vi "rsidr_core_global.vi"() -> ()   [LabVIEW 2020, in "Rohde&Schwarz RTx Oscilloscopes.lvlib"] (continued)
 "Access"=0, "Range Table"="", "Read Callback"="", "Write Callback"="", "Supported Models"="", "Instrument Options"="", "Flags"=0, "Help"="Return the time of the first sample of the indicated waveform.\n\nAvailable Repeated Capabilities:\nChannel: CH0, CH1, CH2, CH3, CH4, CHExt\r\n\nRemote-control command(s):\nCHANnel<m>:DATA:ENVelope:XORigin?"}, {"Level"=3, "Class Only"=FALSE, "Identifier"="RSRTX_ATTR_ENVELOPE_WAVEFORM_CONVERSION_X_INCREMENT", "Descriptive Name"="Envelope Waveform Conversion X Increment", "Data Type"=1, "Command"="CHAN{Channel}:DATA:ENV:XINC?", "Access"=0, "Range Table"="", "Read Callback"="", "Write Callback"="", "Supported Models"="", "Instrument Options"="", "Flags"=0, "Help"="Return the time difference between two adjacent samples of the indicated waveform.\n\nAvailable Repeated Capabilities:\nChannel: CH0, CH1, CH2, CH3, CH4, CHExt\r\n\nRemote-control command(s):\nCHANnel<m>:DATA:ENVelope:XINCrement?"}, {"Level"=3, "Class Only"=FALSE, "Identifier"="RSRTX_ATTR_ENVELOPE_WAVEFORM_CONVERSION_Y_START", "Descriptive Name"="Envelope Waveform Conversion Y Start", "Data Type"=1, "Command"="CHAN{Channel}:DATA:ENV:YOR?", "Access"=0, "Range Table"="", "Read Callback"="", "Write Callback"="", "Supported Models"="", "Instrument Options"="", "Flags"=0, "Help"="Return the voltage value for binary value 0 of the indicated waveform.\n\nAvailable Repeated Capabilities:\nChannel: CH0, CH1, CH2, CH3, CH4, CHExt\r\n\nRemote-control command(s):\nCHANnel<m>:DATA:ENVelope:YORigin?"}, {"Level"=3, "Class Only"=FALSE, "Identifier"="RSRTX_ATTR_ENVELOPE_WAVEFORM_CONVERSION_Y_INCREMENT", "Descriptive Name"="Envelope Waveform Conversion Y Increment", "Data Type"=1, "Command"="CHAN{Channel}:DATA:ENV:YINC?", "Access"=0, "Range Table"="", "Read Callback"="", "Write Callback"="", "Supported Models"="", "Instrument Options"="", "Flags"=0, "Help"="Return the voltage value per bit of the indicated waveform.\n\nAvailable Repeated Capabilities:\nChannel: CH0, CH1, CH2, CH3, CH4, CHExt\r\n\nRemote-control command(s):\nCHANnel<m>:DATA:ENVelope:YINCrement?"}, {"Level"=3, "Class Only"=FALSE, "Identifier"="RSRTX_ATTR_ENVELOPE_WAVEFORM_CONVERSION_Y_RESOLUTION", "Descriptive Name"="Envelope Waveform Conversion Y Resolution", "Data Type"=0, "Command"="CHAN{Channel}:DATA:ENV:YRES?", "Access"=0, "Range Table"="", "Read Callback"="", "Write Callback"="", "Supported Models"="", "Instrument Options"="", "Flags"=0, "Help"="Return the vertical bit resolution of the indicated waveform.\n\nAvailable Repeated Capabilities:\nChannel: CH0, CH1, CH2, CH3, CH4, CHExt\r\n\nRemote-control command(s):\nCHANnel<m>:DATA:ENVelope:YRESolution?"}, {"Level"=2, "Class Only"=TRUE, "Identifier"="", "Descriptive Name"="Math Waveform", "Data Type"=0, "Command"="", "Access"=0, "Range Table"="", "Read Callback"="", "Write Callback"="", "Supported Models"="", "Instrument Options"="", "Flags"=0, "Help"="Acquires waveform data."}, {"Level"=2, "Class Only"=TRUE, "Identifier"="", "Descriptive Name"="Math Waveform Conversion", "Data Type"=0, "Command"="", "Access"=0, "Range Table"="", "Read Callback"="", "Write Callback"="", "Supported Models"="", "Instrument Options"="", "Flags"=0, "Help"="Attributes for conversion of math waveform data."}, {"Level"=3, "Class Only"=FALSE, "Identifier"="RSRTX_ATTR_MATH_WAVEFORM_CONVERSION_X_START", "Descriptive Name"="Math Waveform Conversion X Start", "Data Type"=1, "Command"="CALC:MATH{Math}:DATA:XOR?", "Access"=0, "Range Table"="", "Read Callback"="", "Write Callback"="", "Supported Models"="RTM|RTA", "Instrument Options"="", "Flags"=0, "Help"="Return the time of the first sample of the indicated waveform.\n\nAvailable Repeated Capabilities:\nMath: MA1, MA2, MA3, MA4, MA5\r\n\nRemote-control command(s):\nCALCulate:MATH<m>:DATA:XORigin?"}, {"Level"=3, "Class Only"=FALSE, "Identifier"="RSRTX_ATTR_MATH_WAVEFORM_CONVERSION_X_INCREMENT", "Descriptive Name"="Math Waveform Conversion X Increment", "Data Type"=1, "Command"="CALC:MATH{Math}:DATA:XINC?", "Access"=0, "Range Table"="", "Read Callback"="", "Write Callback"="", "Supported Models"="RTM|RTA", "Instrument Options"="", "Flags"=0, "Help"="Return the time difference between two adjacent samples of the indicated waveform.\n\nAvailable Repeated Capabilities:\nMath: MA1, MA2, MA3, MA4, MA5\r\n\nRemote-control command(s):\nCALCulate:MATH<m>:DATA:XINCrement?"}, {"Level"=3, "Class Only"=FALSE, "Identifier"="RSRTX_ATTR_MATH_WAVEFORM_CONVERSION_Y_START", "Descriptive Name"="Math Waveform Conversion Y Start", "Data Type"=1, "Command"="CALC:MATH{Math}:DATA:YOR?", "Access"=0, "Range Table"="", "Read Callback"="", "Write Callback"="", "Supported Models"="RTM|RTA", "Instrument Options"="", "Flags"=0, "Help"="Return the voltage value for binary value 0 of the indicated waveform.\n\nAvailable Repeated Capabilities:\nMath: MA1, MA2, MA3, MA4, MA5\r\n\nRemote-control command(s):\nCALCulate:MATH<m>:DATA:YORigin?"}, {"Level"=3, "Class Only"=FALSE, "Identifier"="RSRTX_ATTR_MATH_WAVEFORM_CONVERSION_Y_INCREMENT", "Descriptive Name"="Math Waveform Conversion Y Increment", "Data Type"=1, "Command"="CALC:MATH{Math}:DATA:YINC?", "Access"=0, "Range Table"="", "Read Callback"="", "Write Callback"="", "Supported Models"="RTM|RTA", "Instrument Options"="", "Flags"=0, "Help"="Return the voltage value per bit of the indicated waveform.\n\nAvailable Repeated Capabilities:\nMath: MA1, MA2, MA3, MA4, MA5\r\n\nRemote-control command(s):\nCALCulate:MATH<m>:DATA:YINCrement?"}, {"Level"=3, "Class Only"=FALSE, "Identifier"="RSRTX_ATTR_MATH_WAVEFORM_CONVERSION_Y_RESOLUTION", "Descriptive Name"="Math Waveform Conversion Y Resolution", "Data Type"=0, "Command"="CALC:MATH{Math}:DATA:YRES?", "Access"=0, "Range Table"="", "Read Callback"="", "Write Callback"="", "Supported Models"="RTM|RTA", "Instrument Options"="", "Flags"=0, "Help"="Return the vertical bit resolution of the indicated waveform.\n\nAvailable Repeated Capabilities:\nMath: MA1, MA2, MA3, MA4, MA5\r\n\nRemote-control command(s):\nCALCulate:MATH<m>:DATA:YRESolution?"}, {"Level"=2, "Class Only"=TRUE, "Identifier"="", "Descriptive Name"="Simple Math Waveform (RTB)", "Data Type"=0, "Command"="", "Access"=0, "Range Table"="", "Read Callback"="", "Write Callback"="", "Supported Models"="", "Instrument Options"="", "Flags"=0, "Help"="Acquires waveform data."}, {"Level"=2, "Class Only"=TRUE, "Identifier"="", "Descriptive Name"="Simple Math Waveform Conversion (RTB)", "Data Type"=0, "Command"="", "Access"=0, "Range Table"="", "Read Callback"="", "Write Callback"="", "Supported Models"="", "Instrument Options"="", "Flags"=0, "Help"="Attributes for conversion of math waveform data."}, {"Level"=3, "Class Only"=FALSE, "Identifier"="RSRTX_ATTR_SIMPLE_MATH_WAVEFORM_CONVERSION_X_START", "Descriptive Name"="Simple Math Waveform Conversion X Start", "Data Type"=1, "Command"="CALC:QMAT:DATA:XOR?", "Access"=0, "Range Table"="", "Read Callback"="", "Write Callback"="", "Supported Models"="RTB", "Instrument Options"="", "Flags"=0, "Help"="Return the time of the first sample of the indicated waveform.\n\nAvailable Repeated Capabilities:\nNone\n\nRemote-control command(s):\nCALCulate:QMATh:DATA:XORigin?"}, {"Level"=3, "Class Only"=FALSE, "Identifier"="RSRTX_ATTR_SIMPLE_MATH_WAVEFORM_CONVERSION_X_INCREMENT", "Descriptive Name"="Simple Math Waveform Conversion X Increment", "Data Type"=1, "Command"="CALC:QMAT:DATA:XINC?", "Access"=0, "Range Table"="", "Read Callback"="", "Write Callback"="", "Supported Models"="RTB", "Instrument Options"="", "Flags"=0, "Help"="Return the time difference between two adjacent samples of the indicated waveform.\n\nAvailable Repeated Capabilities:\nNone\n\nRemote-control command(s):\nCALCulate:QMATh:DATA:XINCrement?"}, {"Level"=3, "Class Only"=FALSE, "Identifier"="RSRTX_ATTR_SIMPLE_MATH_WAVEFORM_CONVERSION_Y_START", "Descriptive Name"="Simple Math Waveform Conversion Y Start", "Data Type"=1, "Command"="CALC:QMAT:DATA:YOR?", "Access"=0, "Range Table"="", "Read Callback"="", "Write Callback"="", "Supported Models"="RTB", "Instrument Options"="", "Flags"=0, "Help"="Return the voltage value for binary value 0 of the indicated waveform.\n\nAvailable Repeated Capabilities:\nNone\n\nRemote-control command(s):\nCALCulate:QMATh:DATA:YORigin?"}, {"Level"=3, "Class Only"=FALSE, "Identifier"="RSRTX_ATTR_SIMPLE_MATH_WAVEFORM_CONVERSION_Y_INCREMENT", "Descriptive Name"="Simple Math Waveform Conversion Y Increment", "Data Type"=1, "Command"="CALC:QMAT:DATA:YINC?", "Access"=0, "Range Table"="", "Read Callback"="", "Write Callback"="", "Supported Models"="RTB", "Instrument Options"="", "Flags"=0, "Help"="Return the voltage value per bit of the indicated waveform.\n\nAvailable Repeated Capabilities:\nNone\n\nRemote-control command(s):\nCALCulate:QMATh:DATA:YINCrement?"}, {"Level"=3, "Class Only"=FALSE, "Identifier"="RSRTX_ATTR_SIMPLE_MATH_WAVEFORM_CONVERSION_Y_RESOLUTION", "Descriptive Name"="Simple Math Waveform Conversion Y Resolution", "Data Type"=0, "Command"="CALC:QMAT:DATA:YRES?", "Access"=0, "Range Table"="", "Read Callback"="", "Write Callback"="", "Supported Models"="RTB", "Instrument Options"="", "Flags"=0, "Help"="Return the vertical bit resolution of the indicated waveform.\n\nAvailable Repeated Capabilities:\nNone\n\nRemote-control command(s):\nCALCulate:QMATh:DATA:YRESolution?"}, {"Level"=2, "Class Only"=TRUE, "Identifier"="", "Descriptive Name"="Reference Waveform", "Data Type"=0, "Command"="", "Access"=0, "Range Table"="", "Read Callback"="", "Write Callback"="", "Supported Models"="", "Instrument Options"="", "Flags"=0, "Help"="Acquires waveform data."}, {"Level"=2, "Class Only"=TRUE, "Identifier"="", "Descriptive Name"="Reference Waveform Conversion", "Data Type"=0, "Command"="", "Access"=0, "Range Table"="", "Read Callback"="", "Write Callback"="", "Supported Models"="", "Instrument Options"="", "Flags"=0, "Help"="Attributes for conversion of reference waveform data."}, {"Level"=3, "Class Only"=FALSE, "Identifier"="RSRTX_ATTR_REFERENCE_WAVEFORM_CONVERSION_X_START", "Descriptive Name"="Reference Waveform Conversion X Start", "Data Type"=1, "Command"="REFC{ReferenceWfm}:DATA:XOR?", "Access"=0, "Range Table"="", "Read Callback"="", "Write Callback"="", "Supported Models"="", "Instrument Options"="", "Flags"=0, "Help"="Return the time of the first sample of the indicated waveform.\n\nAvailable Repeated Capabilities:\nReferenceWfm: RW1, RW2, RW3, RW4\r\n\nRemote-control command(s):\nREFCurvel<m>:DATA:XORigin?"}, {"Level"=3, "Class Only"=FALSE, "Identifier"="RSRTX_ATTR_REFERENCE_WAVEFORM_CONVERSION_X_INCREMENT", "Descriptive Name"="Reference Waveform Conversion X Increment", "Data Type"=1, "Command"="REFC{ReferenceWfm}:DATA:XINC?", "Access"=0, "Range Table"="", "Read Callback"="", "Write Callback"="", "Supported Models"="", "Instrument Options"="", "Flags"=0, "Help"="Return the time difference between two adjacent samples of the indicated waveform.\n\nAvailable Repeated Capabilities:\nReferenceWfm: RW1, RW2, RW3, RW4\r\n\nRemote-control command(s):\nREFCurve<m>:DATA:XINCrement?"}, {"Level"=3, "Class Only"=FALSE, "Identifier"="RSRTX_ATTR_REFERENCE_WAVEFORM_CONVERSION_Y_START", "Descriptive Name"="Reference Waveform Conversion Y Start", "Data Type"=1, "Command"="REFC{ReferenceWfm}:DATA:YOR?", "Access"=0, "Range Table"="", "Read Callback"="", "Write Callback"="", "Supported Models"="", "Instrument Options"="", "Flags"=0, "Help"="Return the voltage value for binary value 0 of the indicated waveform.\n\nAvailable Repeated Capabilities:\nReferenceWfm: RW1, RW2, RW3, RW4\r\n\nRemote-control command(s):\nREFCurve<m>:DATA:YORigin?"}, {"Level"=3, "Class Only"=FALSE, "Identifier"="RSRTX_ATTR_REFERENCE_WAVEFORM_CONVERSION_Y_INCREMENT", "Descriptive Name"="Reference Waveform Conversion Y Increment", "Data Type"=1, "Command"="REFC{ReferenceWfm}:DATA:YINC?", "Access"=0, "Range Table"="", "Read Callback"="", "Write Callback"="", "Supported Models"="", "Instrument Options"="", "Flags"=0, "Help"="Return the voltage value per bit of the indicated waveform.\n\nAvailable Repeated Capabilities:\nReferenceWfm: RW1, RW2, RW3, RW4\r\n\nRemote-control command(s):\nREFCurve<m>:DATA:YINCrement?"}, {"Level"=3, "Class Only"=FALSE, "Identifier"="RSRTX_ATTR_REFERENCE_WAVEFORM_CONVERSION_Y_RESOLUTION", "Descriptive Name"="Reference Waveform Conversion Y Resolution", "Data Type"=0, "Command"="REFC{ReferenceWfm}:DATA:YRES?", "Access"=0, "Range Table"="", "Read Callback"="", "Write Callback"="", "Supported Models"="", "Instrument Options"="", "Flags"=0, "Help"="Return the vertical bit resolution of the indicated waveform.\n\nAvailable Repeated Capabilities:\nReferenceWfm: RW1, RW2, RW3, RW4\r\n\nRemote-control command(s):\nREFCurve<m>:DATA:YRESolution?"}, {"Level"=2, "Class Only"=TRUE, "Identifier"="", "Descriptive Name"="Mask Data", "Data Type"=0, "Command"="", "Access"=0, "Range Table"="", "Read Callback"="", "Write Callback"="", "Supported Models"="", "Instrument Options"="", "Flags"=0, "Help"="Acquires mask data."}, {"Level"=2, "Class Only"=TRUE, "Identifier"="", "Descriptive Name"="Mask Data Conversion", "Data Type"=0, "Command"="", "Access"=0, "Range Table"="", "Read Callback"="", "Write Callback"="", "Supported Models"="", "Instrument Options"="", "Flags"=0, "Help"="Attributes for conversion of mask data."}, {"Level"=3, "Class Only"=FALSE, "Identifier"="RSRTX_ATTR_MASK_DATA_CONVERSION_X_START", "Descriptive Name"="Mask Data Conversion X Start", "Data Type"=1, "Command"="MASK:DATA:XOR?", "Access"=0, "Range Table"="", "Read Callback"="", "Write Callback"="", "Supported Models"="", "Instrument Options"="", "Flags"=0, "Help"="Return the time of the first sample of the indicated waveform.\n\nAvailable Repeated Capabilities:\nNone\n\nRemote-control command(s):\nMASK:DATA:XORigin?"}, {"Level"=3, "Class Only"=FALSE, "Identifier"="RSRTX_ATTR_MASK_DATA_CONVERSION_X_INCREMENT", "Descriptive Name"="Mask Data Conversion X Increment", "Data Type"=1, "Command"="MASK:DATA:XINC?", "Access"=0, "Range Table"="", "Read Callback"="", "Write Callback"="", "Supported Models"="", "Instrument Options"="", "Flags"=0, "Help"="Return the time difference between two adjacent samples of the indicated waveform.\n\nAvailable Repeated Capabilities:\nNone\n\nRemote-control command(s):\nMASK:DATA:XINCrement?"}, {"Level"=3, "Class Only"=FALSE, "Identifier"="RSRTX_ATTR_MASK_DATA_CONVERSION_Y_START", "Descriptive Name"="Mask Data Conversion Y Start", "Data Type"=1, "Command"="MASK:DATA:YOR?", "Access"=0, "Range Table"="", "Read Callback"="", "Write Callback"="", "Supported Models"="", "Instrument Options"="", "Flags"=0, "Help"="Return the voltage value for binary value 0 of the indicated waveform.\n\nAvailable Repeated Capabilities:\nNone\n\nRemote-control command(s):\nMASK:DATA:YORigin?"}, {"Level"=3, "Class Only"=FALSE, "Identifier"="RSRTX_ATTR_MASK_DATA_CONVERSION_Y_INCREMENT", "Descriptive Name"="Mask Data Conversion Y Increment", "Data Type"=1, "Command"="MASK:DATA:YINC?", "Access"=0, "Range Table"="", "Read Callback"="", "Write Callback"="", "Supported Models"="", "Instrument Options"="", "Flags"=0, "Help"="Return the voltage value per bit of the indicated waveform.\n\nAvailable Repeated Capabilities:\nNone\n\nRemote-control command(s):\nMASK:DATA:YINCrement?"}, {"Level"=3, "Class Only"=FALSE, "Identifier"="RSRTX_ATTR_MASK_DATA_CONVERSION_Y_RESOLUTION", "Descriptive Name"="Mask Data Conversion Y Resolution", "Data Type"=0, "Command"="MASK:DATA:YRES?", "Access"=0, "Range Table"="", "Read Callback"="", "Write Callback"="", "Supported Models"="", "Instrument Options"="", "Flags"=0, "Help"="Return the vertical bit resolution of the indicated waveform.\n\nAvailable Repeated Capabilities:\nNone\n\nRemote-control command(s):\nMASK:DATA:YRESolution?"}, {"Level"=2, "Class Only"=TRUE, "Identifier"="", "Descriptive Name"="Logic Data", "Data Type"=0, "Command"="", "Access"=0, "Range Table"="", "Read Callback"="", "Write Callback"="", "Supported Models"="", "Instrument Options"="", "Flags"=0, "Help"="Acquires logic data."}, {"Level"=2, "Class Only"=TRUE, "Identifier"="", "Descriptive Name"="Logic Data Conversion", "Data Type"=0, "Command"="", "Access"=0, "Range Table"="", "Read Callback"="", "Write Callback"="", "Supported Models"="", "Instrument Options"="", "Flags"=0, "Help"="Attributes for conversion of logic data."}, {"Level"=3, "Class Only"=FALSE, "Identifier"="RSRTX_ATTR_LOGIC_DATA_CONVERSION_X_START", "Descriptive Name"="Logic Data Conversion X Start", "Data Type"=1, "Command"="LOG{Logic}:DATA:XOR?", "Access"=0, "Range Table"="", "Read Callback"="", "Write Callback"="", "Supported Models"="", "Instrument Options"="", "Flags"=0, "Help"="Return the time of the first sample of the indicated waveform.\n\nAvailable Repeated Capabilities:\nLogic: Logic1, Logic2\r\n\nRemote-control command(s):\nLOGic<p>:DATA:XORigin?"}, {"Level"=3, "Class Only"=FALSE, "Identifier"="RSRTX_ATTR_LOGIC_DATA_CONVERSION_X_INCREMENT", "Descriptive Name"="Logic Data Conversion X Increment", "Data Type"=1, "Command"="LOG{Logic}:DATA:XINC?", "Access"=0, "Range Table"="", "Read Callback"="", "Write Callback"="", "Supported Models"="", "Instrument Options"="", "Flags"=0, "Help"="Return the time difference between two adjacent samples of the indicated waveform.\n\nAvailable Repeated Capabilities:\nLogic: Logic1, Logic2\r\n\nRemote-control command(s):\nLOGic<p>:DATA:XINCrement?"}, {"Level"=3, "Class Only"=FALSE, "Identifier"="RSRTX_ATTR_LOGIC_DATA_CONVERSION_Y_START", "Descriptive Name"="Logic Data Conversion Y Start", "Data Type"=1, "Command"="LOG{Logic}:DATA:YOR?", "Access"=0, "Range Table"="", "Read Callback"="", "Write Callback"="", "Supported Models"="", "Instrument Options"="", "Flags"=0, "Help"="Return the voltage value for binary value 0 of the indicated waveform.\n\nAvailable Repeated Capabilities:\nLogic: Logic1, Logic2\r\n\nRemote-control command(s):\nLOGic<p>:DATA:YORigin?"}, {"Level"=3, "Class Only"=FALSE, "Identifier"="RSRTX_ATTR_LOGIC_DATA_CONVERSION_Y_INCREMENT", "Descriptive Name"="Logic Data Conversion Y Increment", "Data Type"=1, "Command"="LOG{Logic}:DATA:YINC?", "Access"=0, "Range Table"="", "Read Callback"="", "Write Callback"="", "Supported Models"="", "Instrument Options"="", "Flags"=0, "Help"="Return the voltage value per bit of the indicated waveform.\n\nAvailable Repeated Capabilities:\nLogic: Logic1, Logic2\r\n\nRemote-control command(s):\nLOGic<p>:DATA:YINCrement?"}, {"Level"=3, "Class Only"=FALSE, "Identifier"="RSRTX_ATTR_LOGIC_DATA_CONVERSION_Y_RESOLUTION", "Descriptive Name"="Logic Data Conversion Y Resolution", "Data Type"=0, "Command"="LOG{Logic}:DATA:YRES?", "Access"=0, "Range Table"="", "Read Callback"="", "Write Callback"="", "Supported Models"="", "Instrument Options"="", "Flags"=0, "Help"="Return the vertical bit resolution of the indicated waveform.\n\nAvailable Repeated Capabilities:\nLogic: Logic1, Logic2\r\n\nRemote-control command(s):\nLOGic<p>:DATA:YRESolution?"}, {"Level"=2, "Class Only"=TRUE, "Identifier"="", "Descriptive Name"="Digital Data", "Data Type"=0, "Command"="", "Access"=0, "Range Table"="", "Read Callback"="", "Write Callback"="", "Supported Models"="", "Instrument Options"="", "Flags"=0, "Help"="Acquires digital data."}, {"Level"=3, "Class Only"=FALSE, "Identifier"="RSRTX_ATTR_DIGITAL_WAVEFORM_SAMPLES", "Descriptive Name"="Digital Waveform Samples", "Data Type"=0, "Command"="DIG{Digital}:DATA:POIN?", "Access"=0, "Range Table"="", "Read Callback"="", "Write Callback"="", "Supported Models"="", "Instrument Options"="", "Flags"=0, "Help"="Returns the number of returned samples for the selected range.\n\nAvailable Repeated Capabilities:\nDigital: D0, D1, D2, D3, D4, D5, D6, D7, D8, D9, D10, D11, D12, D13, D14, D15\r\n\nRemote-control command(s):\nDIGital<m>:DATA:POINts?"}, {"Level"=2, "Class Only"=TRUE, "Identifier"="", "Descriptive Name"="Digital Data Conversion", "Data Type"=0, "Command"="", "Access"=0, "Range Table"="", "Read Callback"="", "Write Callback"="", "Supported Models"="", "Instrument Options"="", "Flags"=0, "Help"="Attributes for conversion of digital data."}, {"Level"=3, "Class Only"=FALSE, "Identifier"="RSRTX_ATTR_DIGITAL_DATA_CONVERSION_X_START", "Descriptive Name"="Digital Data Conversion X Start", "Data Type"=1, "Command"="DIG{Digital}:DATA:XOR?", "Access"=0, "Range Table"="", "Read Callback"="", "Write Callback"="", "Supported Models"="", "Instrument Options"="", "Flags"=0, "Help"="Return the time of the first sample of the indicated waveform.\n\nAvailable Repeated Capabilities:\nDigital: D0, D1, D2, D3, D4, D5, D6, D7, D8, D9, D10, D11, D12, D13, D14, D15\r\n\nRemote-control command(s):\nDIGital<m>:DATA:XORigin?"}, {"Level"=3, "Class Only"=FALSE, "Identifier"="RSRTX_ATTR_DIGITAL_DATA_CONVERSION_X_INCREMENT", "Descriptive Name"="Digital Data Conversion X Increment", "Data Type"=1, "Command"="DIG{Digital}:DATA:XINC?", "Access"=0, "Range Table"="", "Read Callback"="", "Write Callback"="", "Supported Models"="", "Instrument Options"="", "Flags"=0, "Help"="Return the time difference between two adjacent samples of the indicated waveform.\n\nAvailable Repeated Capabilities:\nDigital: D0, D1, D2, D3, D4, D5, D6, D7, D8, D9, D10, D11, D12, D13, D14, D15\r\n\nRemote-control command(s):\nDIGital<m>:DATA:XINCrement?"}, {"Level"=3, "Class Only"=FALSE, "Identifier"="RSRTX_ATTR_DIGITAL_DATA_CONVERSION_Y_START", "Descriptive Name"="Digital Data Conversion Y Start", "Data Type"=1, "Command"="DIG{Digital}:DATA:YOR?", "Access"=0, "Range Table"="", "Read Callback"="", "Write Callback"="", "Supported Models"="", "Instrument Options"="", "Flags"=0, "Help"="Return the voltage value for binary value 0 of the indicated waveform.\n\nAvailable Repeated Capabilities:\nDigital: D0, D1, D2, D3, D4, D5, D6, D7, D8, D9, D10, D11, D12, D13, D14, D15\r\n\nRemote-control command(s):\nDIGital<m>:DATA:YORigin?"}, {"Level"=3, "Class Only"=FALSE, "Identifier"="RSRTX_ATTR_DIGITAL_DATA_CONVERSION_Y_INCREMENT", "Descriptive Name"="Digital Data Conversion Y Increment", "Data Type"=1, "Command"="DIG{Digital}:DATA:YINC?", "Access"=0, "Range Table"="", "Read Callback"="", "Write Callback"="", "Supported Models"="", "Instrument Options"="", "Flags"=0, "Help"="Return the voltage value per bit of the indicated waveform.\n\nAvailable Repeated Capabilities:\nDigital: D0, D1, D2, D3, D4, D5, D6, D7, D8, D9, D10, D11, D12, D13, D14, D15\r\n\nRemote-control command(s):\nDIGital<m>:DATA:YINCrement?"}, {"Level"=3, "Class Only"=FALSE, "Identifier"="RSRTX_ATTR_DIGITAL_DATA_CONVERSION_Y_RESOLUTION", "Descriptive Name"="Digital Data Conversion Y Resolution", "Data Type"=0, "Command"="DIG{Digital}:DATA:YRES?", "Access"=0, "Range Table"="", "Read Callback"="", "Write Callback"="", "Supported Models"="", "Instrument Options"="", "Flags"=0, "Help"="Return the vertical bit resolution of the indicated waveform.\n\nAvailable Repeated Capabilities:\nDigital: D0, D1, D2, D3, D4, D5, D6, D7, D8, D9, D10, D11, D12, D13, D14, D15\r\n\nRemote-control command(s):\nDIGital<m>:DATA:YRESolution?"}, {"Level"=2, "Class Only"=TRUE, "Identifier"="", "Descriptive Name"="Spectrum Data", "Data Type"=0, "Command"="", "Access"=0, "Range Table"="", "Read Callback"="", "Write Callback"="", "Supported Models"="", "Instrument Options"="", "Flags"=0, "Help"="Acquires spectrum data."}, {"Level"=3, "Class Only"=FALSE, "Identifier"="RSRTX_ATTR_SPECTRUM_WAVEFORM_SAMPLES", "Descriptive Name"="Spectrum Waveform Samples", "Data Type"=0, "Command"="SPEC:WAV:SPEC:DATA:POIN?", "Access"=0, "Range Table"="", "Read Callback"="", "Write Callback"="", "Supported Models"="", "Instrument Options"="", "Flags"=0, "Help"="Returns the number of data samples that are returned with SPECtrum:WAVeform:SPECtrum:DATA.\n\nAvailable Repeated Capabilities:\nNone\n\nRemote-control command(s):\nSPECtrum:WAVeform:SPECtrum:DATA:POINts?"}, {"Level"=3, "Class Only"=TRUE, "Identifier"="", "Descriptive Name"="Minimum", "Data Type"=0, "Command"="", "Access"=0, "Range Table"="", "Read Callback"="", "Write Callback"="", "Supported Models"="", "Instrument Options"="", "Flags"=0, "Help"="Acquires spectrum minimum data."}, {"Level"=4, "Class Only"=FALSE, "Identifier"="RSRTX_ATTR_SPECTRUM_MINIMUM_WAVEFORM_SAMPLES", "Descriptive Name"="Spectrum Minimum Waveform Samples", "Data Type"=0, "Command"="SPEC:WAV:MIN:DATA:POIN?", "Access"=0, "Range Table"="", "Read Callback"="", "Write Callback"="", "Supported Models"="", "Instrument Options"="", "Flags"=0, "Help"="Returns the number of data samples that are returned with SPECtrum:WAVeform:MINimum:DATA.\n\nAvailable Repeated Capabilities:\nNone\n\nRemote-control command(s):\nSPECtrum:WAVeform:MINimum:DATA:POINts?"}, {"Level"=3, "Class Only"=TRUE, "Identifier"="", "Descriptive Name"="Maximum", "Data Type"=0, "Command"="", "Access"=0, "Range Table"="", "Read Callback"="", "Write Callback"="", "Supported Models"="", "Instrument Options"="", "Flags"=0, "Help"="Acquires spectrum maximum data."}, {"Level"=4, "Class Only"=FALSE, "Identifier"="RSRTX_ATTR_SPECTRUM_MAXIMUM_WAVEFORM_SAMPLES", "Descriptive Name"="Spectrum Maximum Waveform Samples", "Data Type"=0, "Command"="SPEC:WAV:MAX:DATA:POIN?", "Access"=0, "Range Table"="", "Read Callback"="", "Write Callback"="", "Supported Models"="", "Instrument Options"="", "Flags"=0, "Help"="Returns the number of data samples that are returned with SPECtrum:WAVeform:xxx:DATA for the indicated waveform.\n\nAvailable Repeated Capabilities:\nNone\n\nRemote-control command(s):\nSPECtrum:WAVeform:MAXimum:DATA:POINts?"}, {"Level"=3, "Class Only"=TRUE, "Identifier"="", "Descriptive Name"="Average", "Data Type"=0, "Command"="", "Access"=0, "Range Table"="", "Read Callback"="", "Write Callback"="", "Supported Models"="", "Instrument Options"="", "Flags"=0, "Help"="Acquires spectrum average data."}, {"Level"=4, "Class Only"=FALSE, "Identifier"="RSRTX_ATTR_SPECTRUM_AVERAGE_WAVEFORM_SAMPLES", "Descriptive Name"="Spectrum Average Waveform Samples", "Data Type"=0, "Command"="SPEC:WAV:AVER:DATA:POIN?", "Access"=0, "Range Table"="", "Read Callback"="", "Write Callback"="", "Supported Models"="", "Instrument Options"="", "Flags"=0, "Help"="Returns the number of data samples that are returned with SPECtrum:WAVeform:xxx:DATA for the indicated waveform.\n\nAvailable Repeated Capabilities:\nNone\n\nRemote-control command(s):\nSPECtrum:WAVeform:AVERage:DATA:POINts?"}, {"Level"=2, "Class Only"=TRUE, "Identifier"="", "Descriptive Name"="Spectrum Data Conversion", "Data Type"=0, "Command"="", "Access"=0, "Range Table"="", "Read Callback"="", "Write Callback"="", "Supported Models"="", "Instrument Options"="", "Flags"=0, "Help"="Attributes for conversion of spectrum data."}, {"Level"=3, "Class Only"=FALSE, "Identifier"="RSRTX_ATTR_SPECTRUM_DATA_CONVERSION_X_START", "Descriptive Name"="Spectrum Data Conversion X Start", "Data Type"=1, "Command"="SPEC:WAV:SPEC:DATA:XOR?", "Access"=0, "Range Table"="", "Read Callback"="", "Write Callback"="", "Supported Models"="", "Instrument Options"="", "Flags"=0, "Help"="Returns the frequency of the first sample of the indicated waveform.\n\nAvailable Repeated Capabilities:\nNone\n\nRemote-control command(s):\nSPECtrum:WAVeform:SPECtrum:DATA:XORigin?"}, {"Level"=3, "Class Only"=FALSE, "Identifier"="RSRTX_ATTR_SPECTRUM_DATA_CONVERSION_X_INCREMENT", "Descriptive Name"="Spectrum Data Conversion X Increment", "Data Type"=1, "Command"="SPEC:WAV:SPEC:DATA:XINC?", "Access"=0, "Range Table"="", "Read Callback"="", "Write Callback"="", "Supported Models"="", "Instrument Options"="", "Flags"=0, "Help"="Return the level difference between two adjacent samples of the indicated waveform.\n\nAvailable Repeated Capabilities:\nNone\n\nRemote-control command(s):\nSPECtrum:WAVeform:SPECtrum:DATA:XINCrement?"}, {"Level"=3, "Class Only"=FALSE, "Identifier"="RSRTX_ATTR_SPECTRUM_DATA_CONVERSION_Y_START", "Descriptive Name"="Spectrum Data Conversion Y Start", "Data Type"=1, "Command"="SPEC:WAV:SPEC:DATA:YOR?", "Access"=0, "Range Table"="", "Read Callback"="", "Write Callback"="", "Supported Models"="", "Instrument Options"="", "Flags"=0, "Help"="Returns the vertical bit resolution of the indicated waveform.\n\nAvailable Repeated Capabilities:\nNone\n\nRemote-control command(s):\nSPECtrum:WAVeform:SPECtrum:DATA:YORigin?"}, {"Level"=3, "Class Only"=FALSE, "Identifier"="RSRTX_ATTR_SPECTRUM_DATA_CONVERSION_Y_INCREMENT", "Descriptive Name"="Spectrum Data Conversion Y Increment", "Data Type"=1, "Command"="SPEC:WAV:SPEC:DATA:YINC?", "Access"=0, "Range Table"="", "Read Callback"="", "Write Callback"="", "Supported Models"="", "Instrument Options"="", "Flags"=0, "Help"="Returns the voltage value per bit of the indicated waveform.\n\nAvailable Repeated Capabilities:\nNone\n\nRemote-control command(s):\nSPECtrum:WAVeform:SPECtrum:DATA:YINCrement?"}, {"Level"=3, "Class Only"=FALSE, "Identifier"="RSRTX_ATTR_SPECTRUM_DATA_CONVERSION_Y_RESOLUTION", "Descriptive Name"="Spectrum Data Conversion Y Resolution", "Data Type"=0, "Command"="SPEC:WAV:SPEC:DATA:YRES?", "Access"=0, "Range Table"="", "Read Callback"="", "Write Callback"="", "Supported Models"="", "Instrument Options"="", "Flags"=0, "Help"="Returns the vertical bit resolution of the indicated waveform.\n\nAvailable Repeated Capabilities:\nNone\n\nRemote-control command(s):\nSPECtrum:WAVeform:SPECtrum:DATA:YRESolution?"}, {"Level"=3, "Class Only"=TRUE, "Identifier"="", "Descriptive Name"="Minimum", "Data Type"=0, "Command"="", "Access"=0, "Range Table"="", "Read Callback"="", "Write Callback"="", "Supported Models"="", "Instrument Options"="", "Flags"=0, "Help"="Attributes for conversion of spectrum minimum data."}, {"Level"=4, "Class Only"=FALSE, "Identifier"="RSRTX_ATTR_SPECTRUM_MINIMUM_DATA_CONVERSION_X_START", "Descriptive Name"="Spectrum Minimum Data Conversion X Start", "Data Type"=1, "Command"="SPEC:WAV:MIN:DATA:XOR?", "Access"=0, "Range Table"="", "Read Callback"="", "Write Callback"="", "Supported Models"="", "Instrument Options"="", "Flags"=0, "Help"="Returns the frequency of the first sample of the indicated waveform.\n\nAvailable Repeated Capabilities:\nNone\n\nRemote-control command(s):\nSPECtrum:WAVeform:MINimum:DATA:XORigin?"}, {"Level"=4, "Class Only"=FALSE, "Identifier"="RSRTX_ATTR_SPECTRUM_MINIMUM_DATA_CONVERSION_X_INCREMENT", "Descriptive Name"="Spectrum Minimum Data Conversion X Increment", "Data Type"=1, "Command"="SPEC:WAV:MIN:DATA:XINC?", "Access"=0, "Range Table"="", "Read Callback"="", "Write Callback"="", "Supported Models"="", "Instrument Options"="", "Flags"=0, "Help"="Return the level difference between two adjacent samples of the indicated waveform.\n\nAvailable Repeated Capabilities:\nNone\n\nRemote-control command(s):\nSPECtrum:WAVeform:MINimum:DATA:XINCrement?"}, {"Level"=4, "Class Only"=FALSE, "Identifier"="RSRTX_ATTR_SPECTRUM_MINIMUM_DATA_CONVERSION_Y_START", "Descriptive Name"="Spectrum Minimum Data Conversion Y Start", "Data Type"=1, "Command"="SPEC:WAV:MIN:DATA:YOR?", "Access"=0, "Range Table"="", "Read Callback"="", "Write Callback"="", "Supported Models"="", "Instrument Options"="", "Flags"=0, "Help"="Returns the vertical bit resolution of the indicated waveform.\n\nAvailable Repeated Capabilities:\nNone\n\nRemote-control command(s):\nSPECtrum:WAVeform:MINimum:DATA:YORigin?"}, {"Level"=4, "Class Only"=FALSE, "Identifier"="RSRTX_ATTR_SPECTRUM_MINIMUM_DATA_CONVERSION_Y_INCREMENT", "Descriptive Name"="Spectrum Minimum Data Conversion Y Increment", "Data Type"=1, "Command"="SPEC:WAV:MIN:DATA:YINC?", "Access"=0, "Range Table"="", "Read Callback"="", "Write Callback"="", "Supported Models"="", "Instrument Options"="", "Flags"=0, "Help"="Returns the voltage value per bit of the indicated waveform.\n\nAvailable Repeated Capabilities:\nNone\n\nRemote-control command(s):\nSPECtrum:WAVeform:MINimum:DATA:YINCrement?"}, {"Level"=4, "Class Only"=FALSE, "Identifier"="RSRTX_ATTR_SPECTRUM_MINIMUM_DATA_CONVERSION_Y_RESOLUTION", "Descriptive Name"="Spectrum Minimum Data Conversion Y Resolution", "Data Type"=0, "Command"="SPEC:WAV:MIN:DATA:YRES?", "Access"=0, "Range Table"="", "Read Callback"="", "Write Callback"="", "Supported Models"="", "Instrument Options"="", "Flags"=0, "Help"="Returns the vertical bit resolution of the indicated waveform.\n\nAvailable Repeated Capabilities:\nNone\n\nRemote-control command(s):\nSPECtrum:WAVeform:MINimum:DATA:YRESolution?"}, {"Level"=3, "Class Only"=TRUE, "Identifier"="", "Descriptive Name"="Maximum", "Data Type"=0, "Command"="", "Access"=0, "Range Table"="", "Read Callback"="", "Write Callback"="", "Supported Models"="", "Instrument Options"="", "Flags"=0, "Help"="Attributes for conversion of spectrum maximum data."}, {"Level"=4, "Class Only"=FALSE, "Identifier"="RSRTX_ATTR_SPECTRUM_MAXIMUM_DATA_CONVERSION_X_START", "Descriptive Name"="Spectrum Maximum Data Conversion X Start", "Data Type"=1, "Command"="SPEC:WAV:MAX:DATA:XOR?", "Access"=0, "Range Table"="", "Read Callback"="", "Write Callback"="", "Supported Models"="", "Instrument Options"="", "Flags"=0, "Help"="Returns the frequency of the first sample of the indicated waveform.\n\nAvailable Repeated Capabilities:\nNone\n\nRemote-control command(s):\nSPECtrum:WAVeform:MAXimum:DATA:XORigin?"}, {"Level"=4, "Class Only"=FALSE, "Identifier"="RSRTX_ATTR_SPECTRUM_MAXIMUM_DATA_CONVERSION_X_INCREMENT", "Descriptive Name"="Spectrum Maximum Data Conversion X Increment", "Data Type"=1, "Command"="SPEC:WAV:MAX:DATA:XINC?", "Access"=0, "Range Table"="", "Read Callback"="", "Write Callback"="", "Supported Models"="", "Instrument Options"="", "Flags"=0, "Help"="Return the level difference between two adjacent samples of the indicated waveform.\n\nAvailable Repeated Capabilities:\nNone\n\nRemote-control command(s):\nSPECtrum:WAVeform:MAXimum:DATA:XINCrement?"}, {"Level"=4, "Class Only"=FALSE, "Identifier"="RSRTX_ATTR_SPECTRUM_MAXIMUM_DATA_CONVERSION_Y_START", "Descriptive Name"="Spectrum Maximum Data Conversion Y Start", "Data Type"=1, "Command"="SPEC:WAV:MAX:DATA:YOR?", "Access"=0, "Range Table"="", "Read Callback"="", "Write Callback"="", "Supported Models"="", "Instrument Options"="", "Flags"=0, "Help"="Returns the vertical bit resolution of the indicated waveform.\n\nAvailable Repeated Capabilities:\nNone\n\nRemote-control command(s):\nSPECtrum:WAVeform:MAXimum:DATA:YORigin?"}, {"Level"=4, "Class Only"=FALSE, "Identifier"="RSRTX_ATTR_SPECTRUM_MAXIMUM_DATA_CONVERSION_Y_INCREMENT", "Descriptive Name"="Spectrum Maximum Data Conversion Y Increment", "Data Type"=1, "Command"="SPEC:WAV:MAX:DATA:YINC?", "Access"=0, "Range Table"="", "Read Callback"="", "Write Callback"="", "Supported Models"="", "Instrument Options"="", "Flags"=0, "Help"="Returns the voltage value per bit of the indicated waveform.\n\nAvailable Repeated Capabilities:\nNone\n\nRemote-control command(s):\nSPECtrum:WAVeform:MAXimum:DATA:YINCrement?"}, {"Level"=4, "Class Only"=FALSE, "Identifier"="RSRTX_ATTR_SPECTRUM_MAXIMUM_DATA_CONVERSION_Y_RESOLUTION", "Descriptive Name"="Spectrum Maximum Data Conversion Y Resolution", "Data Type"=0, "Command"="SPEC:WAV:MAX:DATA:YRES?", "Access"=0, "Range Table"="", "Read Callback"="", "Write Callback"="", "Supported Models"="", "Instrument Options"="", "Flags"=0, "Help"="Returns the vertical bit resolution of the indicated waveform.\n\nAvailable Repeated Capabilities:\nNone\n\nRemote-control command(s):\nSPECtrum:WAVeform:MAXimum:DATA:YRESolution?"}, {"Level"=3, "Class Only"=TRUE, "Identifier"="", "Descriptive Name"="Average", "Data Type"=0, "Command"="", "Access"=0, "Range Table"="", "Read Callback"="", "Write Callback"="", "Supported Models"="", "Instrument Options"="", "Flags"=0, "Help"="Attributes for conversion of spectrum average data."}, {"Level"=4, "Class Only"=FALSE, "Identifier"="RSRTX_ATTR_SPECTRUM_AVERAGE_DATA_CONVERSION_X_START", "Descriptive Name"="Spectrum Average Data Conversion X Start", "Data Type"=1, "Command"="SPEC:WAV:AVER:DATA:XOR?", "Access"=0, "Range Table"="", "Read Callback"="", "Write Callback"="", "Supported Models"="", "Instrument Options"="", "Flags"=0, "Help"="Returns the frequency of the first sample of the indicated waveform.\n\nAvailable Repeated Capabilities:\nNone\n\nRemote-control command(s):\nSPECtrum:WAVeform:AVERage:DATA:XORigin?"}, {"Level"=4, "Class Only"=FALSE, "Identifier"="RSRTX_ATTR_SPECTRUM_AVERAGE_DATA_CONVERSION_X_INCREMENT", "Descriptive Name"="Spectrum Average Data Conversion X Increment", "Data Type"=1, "Command"="SPEC:WAV:AVER:DATA:XINC?", "Access"=0, "Range Table"="", "Read Callback"="", "Write Callback"="", "Supported Models"="", "Instrument Options"="", "Flags"=0, "Help"="Return the level difference between two adjacent samples of the indicated waveform.\n\nAvailable Repeated Capabilities:\nNone\n\nRemote-control command(s):\nSPECtrum:WAVeform:AVERage:DATA:XINCrement?"}, {"Level"=4, "Class Only"=FALSE, "Identifier"="RSRTX_ATTR_SPECTRUM_AVERAGE_DATA_CONVERSION_Y_START", "Descriptive Name"="Spectrum Average Data Conversion Y Start", "Data Type"=1, "Command"="SPEC:WAV:AVER:DATA:YOR?", "Access"=0, "Range Table"="", "Read Callback"="", "Write Callback"="", "Supported Models"="", "Instrument Options"="", "Flags"=0, "Help"="Returns the vertical bit resolution of the indicated waveform.\n\nAvailable Repeated Capabilities:\nNone\n\nRemote-control command(s):\nSPECtrum:WAVeform:AVERage:DATA:YORigin?"}, {"Level"=4, "Class Only"=FALSE, "Identifier"="RSRTX_ATTR_SPECTRUM_AVERAGE_DATA_CONVERSION_Y_INCREMENT", "Descriptive Name"="Spectrum Average Data Conversion Y Increment", "Data Type"=1, "Command"="SPEC:WAV:AVER:DATA:YINC?", "Access"=0, "Range Table"="", "Read Callback"="", "Write Callback"="", "Supported Models"="", "Instrument Options"="", "Flags"=0, "Help"="Returns the voltage value per bit of the indicated waveform.\n\nAvailable Repeated Capabilities:\nNone\n\nRemote-control command(s):\nSPECtrum:WAVeform:AVERage:DATA:YINCrement?"}, {"Level"=4, "Class Only"=FALSE, "Identifier"="RSRTX_ATTR_SPECTRUM_AVERAVE_DATA_CONVERSION_Y_RESOLUTION", "Descriptive Name"="Spectrum Averave Data Conversion Y Resolution", "Data Type"=0, "Command"="SPEC:WAV:AVER:DATA:YRES?", "Access"=0, "Range Table"="", "Read Callback"="", "Write Callback"="", "Supported Models"="", "Instrument Options"="", "Flags"=0, "Help"="Returns the vertical bit resolution of the indicated waveform.\n\nAvailable Repeated Capabilities:\nNone\n\nRemote-control command(s):\nSPECtrum:WAVeform:AVERage:DATA:YRESolution?"}, {"Level"=1, "Class Only"=TRUE, "Identifier"="", "Descriptive Name"="Cursors", "Data Type"=0, "Command"="", "Access"=0, "Range Table"="", "Read Callback"="", "Write Callback"="", "Supported Models"="", "Instrument Options"="", "Flags"=0, "Help"="Cursor measurements determine the results at the current cursor positions. The cursors can be positioned manually or can be configured to follow the peaks of the waveform. Up to four sets of cursors can be configured and displayed. Each set of cursors consists of a pair of horizontal or vertical cursors, or both. Cursors can be coupled so that the initially defined distance is always maintained."}, {"Level"=2, "Class Only"=FALSE, "Identifier"="RSRTX_ATTR_CURSOR_ENABLED", "Descriptive Name"="Cursor Enabled", "Data Type"=3, "Command"="CURS1:STAT", "Access"=2, "Range Table"="", "Read Callback"="", "Write Callback"="", "Supported Models"="", "Instrument Options"="", "Flags"=0, "Help"="Switches the indicated cursor on or off.\n\nAvailable Repeated Capabilities:\nNone\n\nRemote-control command(s):\nCURSor<m>:STATe"}, {"Level"=2, "Class Only"=FALSE, "Identifier"="RSRTX_ATTR_ALL_CURSORS_OFF", "Descriptive Name"="All Cursors Off", "Data Type"=4, "Command"="CURS1:AOFF", "Access"=1, "Range Table"="", "Read Callback"="", "Write Callback"="", "Supported Models"="", "Instrument Options"="", "Flags"=0, "Help"="Switches all cursors off.\n\nAvailable Repeated Capabilities:\nNone\n\nRemote-control command(s):\nCURSor<m>:AOFF"}, {"Level"=2, "Class Only"=FALSE, "Identifier"="RSRTX_ATTR_CURSOR_MEASUREMENT_TYPE", "Descriptive Name"="Cursor Measurement Type", "Data Type"=0, "Command"="CURS1:FUNC", "Access"=2, "Range Table"="rsrtx_rngCursorFunction", 
